vi "HttpGetRequest.vi"() -> ()   [LabVIEW 2025]
doc: "Executes a sample API request, stores the response in a body string, and converts the received JSON data into a 2D array."
uses:
  <vilib>/httpClient/LabVIEWHTTPClient.lvlib
panel:
  out "Table Control":string[][](table)
  out "Output Array":string[][](array[string])
  out "response body":string
  # "Executes a sample api and storing response in body string and converting json data to 2D array"
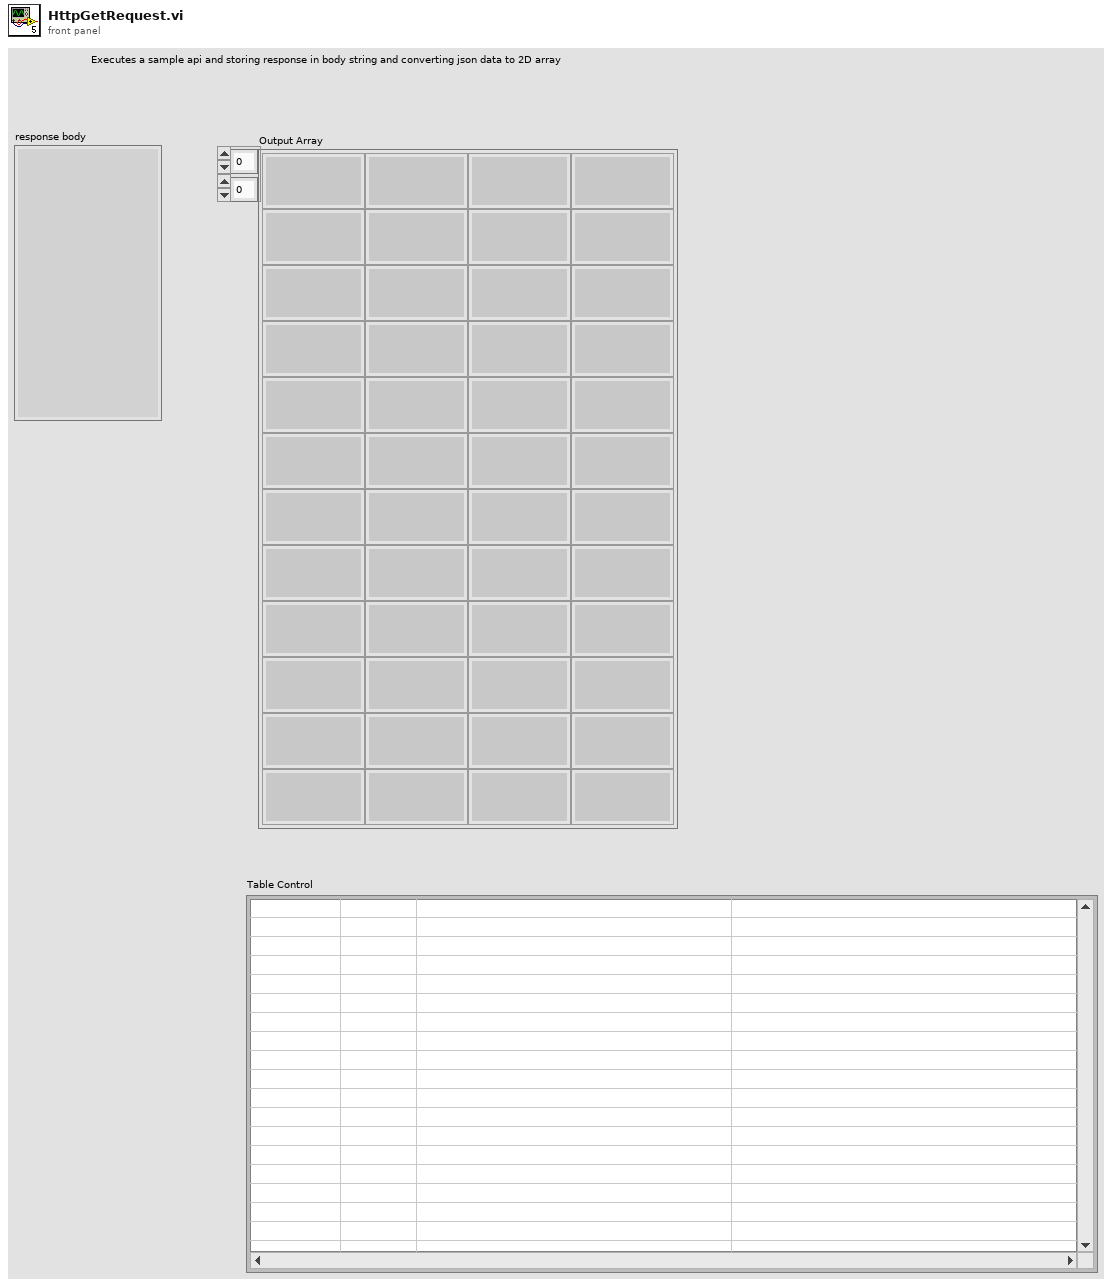
[diagram p1: front panel]
types:
  T1 = cluster{"userId":i32, "id":i32, "title":string, "body":string}[]
  T2 = typedef "LabVIEWHTTPClient.lvlib/ClientHandle.ctl" = refnum<k1>
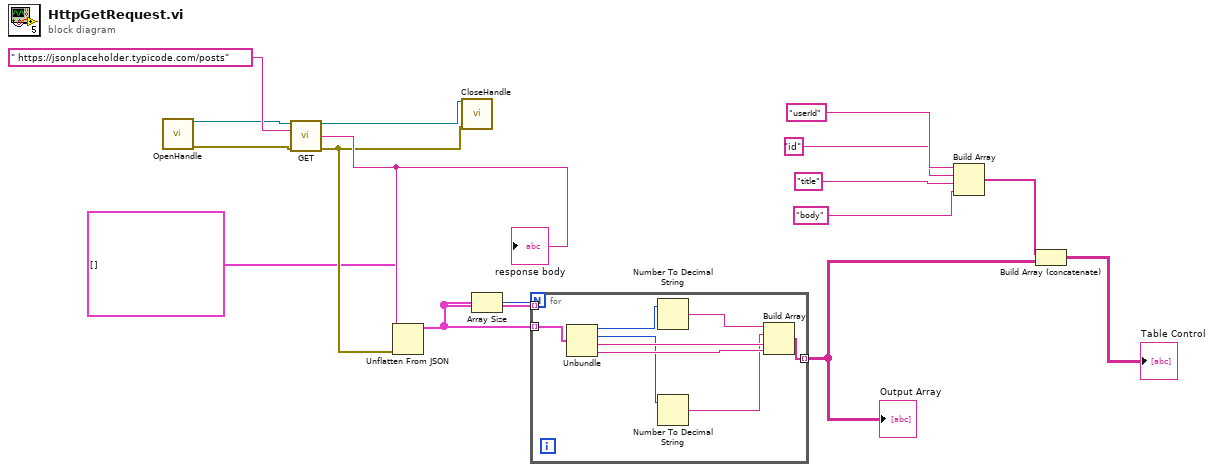
[diagram p0: block diagram]
diagram:
  n1 = call <vilib>:"OpenHandle.vi"() -> ("client handle out"=w14:T2, "error out"=w13:errorcluster)  [unwired: 14 in]
  n2 = call <vilib>:"GET.vi"("client handle"=w14, "url"=" https://jsonplaceholder.typicode.com/posts", "error in (no error)"=w13) -> ("client handle out"=w15:T2, "body"=w12:string, "error out"=w11:errorcluster)  [unwired: 9 in, 1 out]
  "response body" <- w12
  n3 = Unflatten From JSON(JSON string=w12, type and defaults=T1 [], error in (no error)=w11) -> (value=w9:T1)  [unwired: 4 in, 1 out]
  n4 = call <vilib>:"CloseHandle.vi"("client handle"=w15, "error in (no error)"=w11) -> ()  [unwired: 13 in, 1 out]
  n5 = Array Size(array=w9) -> (size(s)=w10:i32)
  n6 = for {
    N: w10 -> [_]
    tunnel: w9 -> [_] mode=indexing
    tunnel: w9 -> [w24] mode=indexing
    tunnel: [w17] -> w7 mode=indexing
    n7 = Unbundle(w24) -> ("userId"=w21:i32, "id"=w19:i32, "title"=w22:string, "body"=w23:string)
    n8 = Number To Decimal String(number=w21) -> (decimal integer string=w20:string)  [unwired: 1 in]
    n9 = Number To Decimal String(number=w19) -> (decimal integer string=w18:string)  [unwired: 1 in]
    n10 = Build Array(w20, w18, w22, w23) -> (w17:string[])
  }
  "Output Array" <- w7
  n11 = Build Array("userId", "id", "title", "body") -> (w1:string[])
  n12 = Build Array (concatenate)(w1, w7) -> (→"Table Control":string[][])
